vi "BeginClimber.vi"() -> (0 "Error Out List":errorcluster[](array[cluster]))   [LabVIEW 2012]
uses:
  <vilib>/Rock Robotics/SystemInterfaces/DIO/FPGA_DIOChannel.ctl
  <vilib>/Rock Robotics/SystemInterfaces/Typedef/FPGA_TypedefAnalogModule.ctl
  <vilib>/Rock Robotics/SystemInterfaces/AI/FPGA_AIChannel.ctl
  <vilib>/Rock Robotics/SystemInterfaces/Typedef/FPGA_TypedefDigitalModule.ctl
  <vilib>/Rock Robotics/SystemInterfaces/DIO/FPGA_DIOPWMChannel.ctl
  <vilib>/Rock Robotics/WPI/MotorControl/WPI_MotorControlOpen Victor.vi
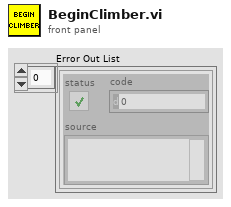
[diagram p1: front panel]
types:
  T1 = typedef "FPGA_TypedefDigitalModule.ctl" = enum16{"Digital Module 1", "Digital Module 2"}
  T2 = typedef "FPGA_DIOChannel.ctl" = enum8{"DIO 1", "DIO 2", "DIO 3", "DIO 4", "DIO 5", "DIO 6", "DIO 7", "DIO 8", "DIO 9", "DIO 10", "DIO 11", "DIO 12", "DIO 13", "DIO 14", "Invalid"}
  T3 = typedef "FPGA_DIOPWMChannel.ctl" = enum8{"PWM 1", "PWM 2", "PWM 3", "PWM 4", "PWM 5", "PWM 6", "PWM 7", "PWM 8", "PWM 9", "PWM 10", "Invalid"}
  T4 = typedef "FPGA_AIChannel.ctl" = enum8{"AI 1", "AI 2", "AI 3", "AI 4", "AI 5", "AI 6", "AI 7", "AI 8", "Invalid"}
  T5 = typedef "FPGA_TypedefAnalogModule.ctl" = enum16{"Analog Module 1", "Analog Module 2"}
  T6 = typedef "WPI_MotorControlDeviceRef.ctl" = cluster{"DeviceStatus":errorcluster, "Type":enum16{"PWM", "CAN"}, "PWM":cluster{"Digital Module":T1, "PWM Channel":T3, "DeadBand":T7}, "CAN":cluster{"Device Number":u8, "Control Mode":T8, "Semaphore":T9, "Max Vout":dbl}, "Invert":bool, "TransformRef":T10, "InvTransformRef":T10}
  T7 = typedef "WPI_PWMDeadband.ctl" = cluster{"Name":string, "maxPositivePwm":i32, "minPositivePwm":i32, "centerPwm":i32, "maxNegativePwm":i32, "minNegativePwm":i32, "angularRange":u16}
  T8 = typedef "WPI_CANJaguar_ControlMode.ctl" = enum8{"Percent VBus", "Current", "Speed", "Position", "Voltage"}
  T9 = typedef "Semaphore RefNum" = refnum<k1>
  T10 = typedef "WPI_PWMTransform_ConPane.ctl" = refnum<vi>
  T11 = typedef "WPI_AnalogChannelDevRef.ctl" = cluster{"DevStatus":errorcluster, "Analog Module":T5, "Analog Channel":T4}
  T12 = typedef "WPI_DigitalInputDevRef.ctl" = cluster{"DevStatus":errorcluster, "DIO Channel":T2, "Digital Module":T1}
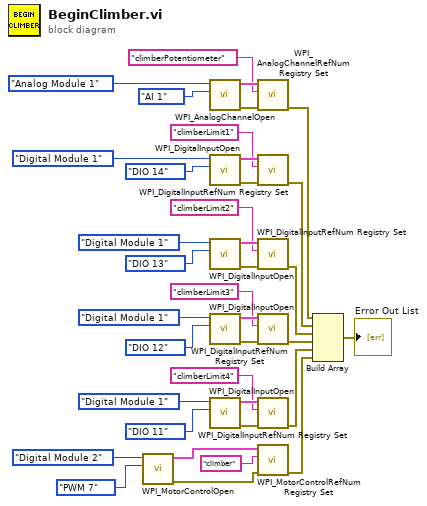
[diagram p0: block diagram]
diagram:
  n1 = call-poly <vilib>:"WPI_MotorControlOpen.vi"("PWM Channel"=FPGA_DIOPWMChannel."PWM 7", "Digital Module (Module 1)"=FPGA_TypedefDigitalModule."Digital Module 2") -> ("error out"=w20:errorcluster, "MotorControlDeviceRef"=w19:T6)  [unwired: 8 in]
  n2 = call <vilib>:"WPI_AnalogChannelOpen.vi"("Analog Channel"=FPGA_AIChannel."AI 1", "Analog Module (Module 1)"=FPGA_TypedefAnalogModule."Analog Module 1") -> ("error out"=w26:errorcluster, "AIDeviceRef"=w25:T11)  [unwired: 8 in]
  n3 = call <vilib>:"WPI_DigitalInputOpen.vi"("DIO Channel"=FPGA_DIOChannel."DIO 14", "Digital Module (Module 1)"=FPGA_TypedefDigitalModule."Digital Module 1") -> ("error out"=w31:errorcluster, "DigitalInputDevRef"=w36:T12)  [unwired: 8 in]
  n4 = call <vilib>:"WPI_DigitalInputOpen.vi"("DIO Channel"=FPGA_DIOChannel."DIO 13", "Digital Module (Module 1)"=FPGA_TypedefDigitalModule."Digital Module 1") -> ("error out"=w30:errorcluster, "DigitalInputDevRef"=w33:T12)  [unwired: 8 in]
  n5 = call <vilib>:"WPI_DigitalInputOpen.vi"("DIO Channel"=FPGA_DIOChannel."DIO 12", "Digital Module (Module 1)"=FPGA_TypedefDigitalModule."Digital Module 1") -> ("error out"=w9:errorcluster, "DigitalInputDevRef"=w11:T12)  [unwired: 8 in]
  n6 = call <vilib>:"WPI_DigitalInputOpen.vi"("DIO Channel"=FPGA_DIOChannel."DIO 11", "Digital Module (Module 1)"=FPGA_TypedefDigitalModule."Digital Module 1") -> ("error out"=w4:errorcluster, "DigitalInputDevRef"=w6:T12)  [unwired: 8 in]
  n7 = call <vilib>:"WPI_AnalogChannelRefNum Registry Set.vi"("error in (no error)"=w26, "refnum name"="climberPotentiometer", "AIDeviceRef"=w25) -> ("error out"=w21:errorcluster)  [unwired: 7 in, 1 out]
  n8 = call <vilib>:"WPI_DigitalInputRefNum Registry Set.vi"("error in (no error)"=w31, "refnum name"="climberLimit1", "DigitalInputDevRef"=w36) -> ("error out"=w27:errorcluster)  [unwired: 7 in, 1 out]
  n9 = call <vilib>:"WPI_DigitalInputRefNum Registry Set.vi"("error in (no error)"=w30, "refnum name"="climberLimit2", "DigitalInputDevRef"=w33) -> ("error out"=w29:errorcluster)  [unwired: 7 in, 1 out]
  n10 = call <vilib>:"WPI_DigitalInputRefNum Registry Set.vi"("error in (no error)"=w9, "refnum name"="climberLimit3", "DigitalInputDevRef"=w11) -> ("error out"=w2:errorcluster)  [unwired: 7 in, 1 out]
  n11 = call <vilib>:"WPI_DigitalInputRefNum Registry Set.vi"("error in (no error)"=w4, "refnum name"="climberLimit4", "DigitalInputDevRef"=w6) -> ("error out"=w1:errorcluster)  [unwired: 7 in, 1 out]
  n12 = call <vilib>:"WPI_MotorControlRefNum Registry Set.vi"("error in (no error)"=w20, "refnum name"="climber", "MotorControlDevRef"=w19) -> ("error out"=w13:errorcluster)  [unwired: 7 in, 1 out]
  n13 = Build Array(w21, w27, w29, w2, w1, w13) -> (→"Error Out List":errorcluster[])
